vi "DAQmx.Dark.Current.SubVI.model.vi"(6 "Data to Send in":u32[](array[numeric])=[1, 2, 4, 8, 16, 32, 64, 128], 7 "Data Pin in":tag="Dev1/port0/line0:7", 9 "Write Pin in":tag="Dev1/port0/line0:7", 10 "Sync Pin in":tag="Dev1/port0/line0:7", 11 "Clear Pin in":tag="Dev1/port0/line0:7") -> ()   [LabVIEW 2020]
uses:
  <vilib>/DAQmx/write.llb/DAQmx Write (Digital U32 1Chan 1Samp).vi
  <vilib>/DAQmx/write.llb/DAQmx Write (Digital Bool 1Line 1Point).vi
  <vilib>/DAQmx/create/channels.llb/DAQmx Create Channel (DO-Digital Output).vi
  <vilib>/DAQmx/miscellaneous.llb/DAQmx Fill In Error Info.vi
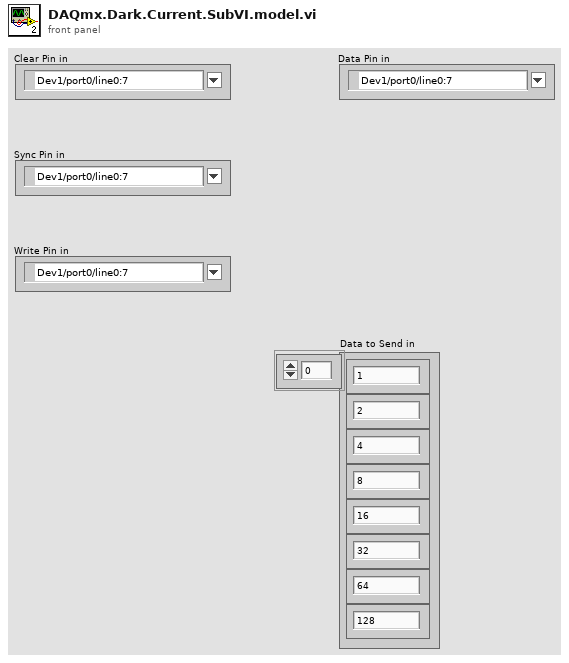
[diagram p1: front panel]
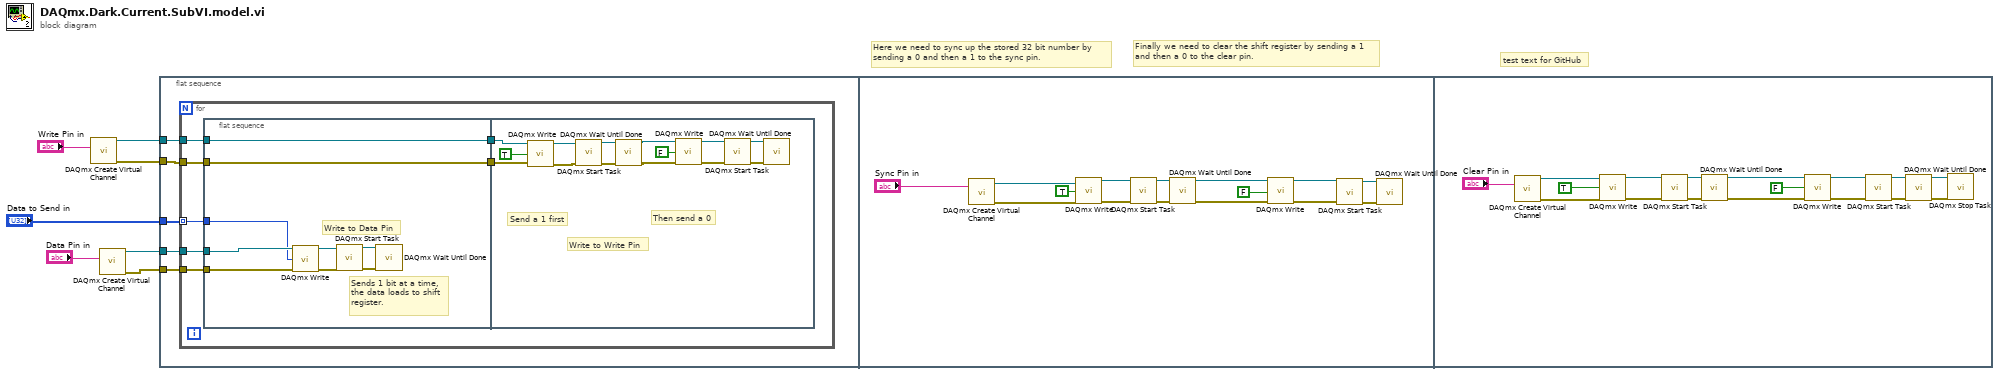
[diagram p0: block diagram]
diagram:
  # "test text for GitHub"
  # "Finally we need to clear the shift register by sending a 1\nand then a 0 to the clear pin."
  # "Here we need to sync up the stored 32 bit number by \nsending a 0 and then a 1 to the sync pin."
  n1 = call-poly <vilib>:"DAQmx Create Virtual Channel.vi"("lines"="Write Pin in") -> ("task out"=w2:refnum<k21>, "error out"=w3:errorcluster)  [unwired: 13 in]
  n2 = call-poly <vilib>:"DAQmx Create Virtual Channel.vi"("lines"="Data Pin in") -> ("task out"=w5:refnum<k21>, "error out"=w6:errorcluster)  [unwired: 13 in]
  n3 = flat-sequence {
    tunnel: w2 -> [w12]
    tunnel: w3 -> [w11]
    tunnel: w5 -> [w10]
    tunnel: w6 -> [w9]
    tunnel: "Data to Send in" -> [w8]
    frame #0 {
      n4 = for {
        tunnel: w12 -> [w19]
        tunnel: w11 -> [w17]
        tunnel: w10 -> [w15]
        tunnel: w9 -> [w14]
        tunnel: w8 -> [w13] mode=indexing
        n5 = flat-sequence {
          tunnel: w19 -> [w28]
          tunnel: [w28] -> w18
          tunnel: w17 -> [w27]
          tunnel: [w27] -> w16
          tunnel: w15 -> [w26]
          tunnel: w14 -> [w25]
          tunnel: w13 -> [w24]
          tunnel: w18 -> [w30]
          tunnel: w16 -> [w29]
          frame #0 {
            # "Sends 1 bit at a time,\nthe data loads to shift\nregister."
            # "Write to Data Pin"
            n6 = call-poly <vilib>:"DAQmx Write.vi"("task/channels in"=w26, "data"=w24, "error in"=w25) -> ("task out"=w22:refnum<k21>, "error out"=w21:errorcluster)  [unwired: 10 in, 1 out]
            n7 = call <vilib>:"DAQmx Start Task.vi"("task/channels in"=w22, "error in"=w21) -> ("task out"=w20:refnum<k21>, "error out"=w23:errorcluster)  [unwired: 12 in]
            n8 = call <vilib>:"DAQmx Wait Until Done.vi"("task/channels in"=w20, "error in"=w23) -> ()  [unwired: 12 in, 2 out]
          }
          frame #1 {
            # "Then send a 0"
            # "Send a 1 first"
            # "Write to Write Pin"
            n9 = call-poly <vilib>:"DAQmx Write.vi"("task/channels in"=w30, "data"=TRUE, "error in"=w29) -> ("task out"=w41:refnum<k21>, "error out"=w40:errorcluster)  [unwired: 10 in, 1 out]
            n10 = call <vilib>:"DAQmx Start Task.vi"("task/channels in"=w41, "error in"=w40) -> ("task out"=w39:refnum<k21>, "error out"=w42:errorcluster)  [unwired: 12 in]
            n11 = call <vilib>:"DAQmx Wait Until Done.vi"("task/channels in"=w39, "error in"=w42) -> ("task out"=w32:refnum<k21>, "error out"=w31:errorcluster)  [unwired: 12 in]
            n12 = call-poly <vilib>:"DAQmx Write.vi"("task/channels in"=w32, "data"=FALSE, "error in"=w31) -> ("task out"=w34:refnum<k21>, "error out"=w33:errorcluster)  [unwired: 10 in, 1 out]
            n13 = call <vilib>:"DAQmx Start Task.vi"("task/channels in"=w34, "error in"=w33) -> ("task out"=w35:refnum<k21>, "error out"=w36:errorcluster)  [unwired: 12 in]
            n14 = call <vilib>:"DAQmx Wait Until Done.vi"("task/channels in"=w35, "error in"=w36) -> ()  [unwired: 12 in, 2 out]
          }
        }
      }
    }
    frame #1 {
      n15 = call-poly <vilib>:"DAQmx Create Virtual Channel.vi"("lines"="Sync Pin in") -> ("task out"=w56:refnum<k21>, "error out"=w52:errorcluster)  [unwired: 13 in]
      n16 = call-poly <vilib>:"DAQmx Write.vi"("task/channels in"=w56, "data"=TRUE, "error in"=w52) -> ("task out"=w53:refnum<k21>, "error out"=w51:errorcluster)  [unwired: 10 in, 1 out]
      n17 = call <vilib>:"DAQmx Start Task.vi"("task/channels in"=w53, "error in"=w51) -> ("task out"=w54:refnum<k21>, "error out"=w50:errorcluster)  [unwired: 12 in]
      n18 = call <vilib>:"DAQmx Wait Until Done.vi"("task/channels in"=w54, "error in"=w50) -> ("task out"=w48:refnum<k21>, "error out"=w47:errorcluster)  [unwired: 12 in]
      n19 = call-poly <vilib>:"DAQmx Write.vi"("task/channels in"=w48, "data"=FALSE, "error in"=w47) -> ("task out"=w44:refnum<k21>, "error out"=w43:errorcluster)  [unwired: 10 in, 1 out]
      n20 = call <vilib>:"DAQmx Start Task.vi"("task/channels in"=w44, "error in"=w43) -> ("task out"=w46:refnum<k21>, "error out"=w45:errorcluster)  [unwired: 12 in]
      n21 = call <vilib>:"DAQmx Wait Until Done.vi"("task/channels in"=w46, "error in"=w45) -> ()  [unwired: 12 in, 2 out]
    }
    frame #2 {
      n22 = call-poly <vilib>:"DAQmx Create Virtual Channel.vi"("lines"="Clear Pin in") -> ("task out"=w68:refnum<k21>, "error out"=w69:errorcluster)  [unwired: 13 in]
      n23 = call-poly <vilib>:"DAQmx Write.vi"("task/channels in"=w68, "data"=TRUE, "error in"=w69) -> ("task out"=w72:refnum<k21>, "error out"=w71:errorcluster)  [unwired: 10 in, 1 out]
      n24 = call <vilib>:"DAQmx Start Task.vi"("task/channels in"=w72, "error in"=w71) -> ("task out"=w74:refnum<k21>, "error out"=w73:errorcluster)  [unwired: 12 in]
      n25 = call <vilib>:"DAQmx Wait Until Done.vi"("task/channels in"=w74, "error in"=w73) -> ("task out"=w66:refnum<k21>, "error out"=w65:errorcluster)  [unwired: 12 in]
      n26 = call-poly <vilib>:"DAQmx Write.vi"("task/channels in"=w66, "data"=FALSE, "error in"=w65) -> ("task out"=w61:refnum<k21>, "error out"=w60:errorcluster)  [unwired: 10 in, 1 out]
      n27 = call <vilib>:"DAQmx Start Task.vi"("task/channels in"=w61, "error in"=w60) -> ("task out"=w63:refnum<k21>, "error out"=w62:errorcluster)  [unwired: 12 in]
      n28 = call <vilib>:"DAQmx Wait Until Done.vi"("task/channels in"=w63, "error in"=w62) -> ("task out"=w59:refnum<k21>, "error out"=w58:errorcluster)  [unwired: 12 in]
      n29 = call <vilib>:"DAQmx Stop Task.vi"("task/channels in"=w59, "error in"=w58) -> ()  [unwired: 12 in, 2 out]
    }
  }
